vi "Post Test End.vi"(8 "error in (no error)":errorcluster, 9 "Test End Error (no error)":errorcluster, 10 "Test End":enum16{"Normal", "User Abort", "Error"}(ring), 11 "Test":T1) -> (0 "error out":errorcluster)   [LabVIEW 2016, in "Hall Effect Library.lvlib"]
uses:
  Hall Effect Library.lvlib
  Public/Controls/Tests.ctl
  Public/Controls/Message Types.ctl
  Global Variables/Communication.vi
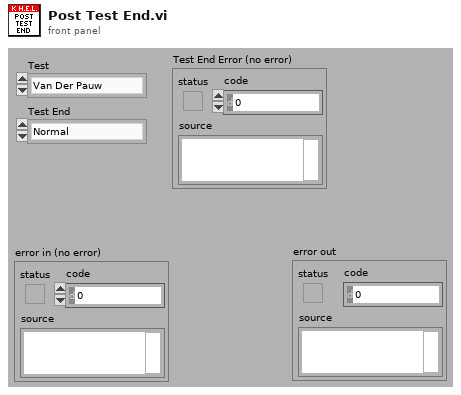
[diagram p1: front panel]
types:
  T1 = typedef "Hall Effect Library.lvlib/Tests.ctl" = enum16{"Van Der Pauw", "Hall Effect", "Bar Sample Resistivity", "Bar Sample Hall ", "6-Contact Sample Resistivity", "6-Contact Sample Hall", "8-Contact Sample Resistivity", "8-Contact Sample Hall", ""}
  T2 = typedef "Hall Effect Library.lvlib/Message Types.ctl" = enum16{"Status", "New Data", "Test End Normal", "Test End User Abort", "Test End Error"}
  T3 = cluster{"Test":T1, "Test End Error (no error)":errorcluster}
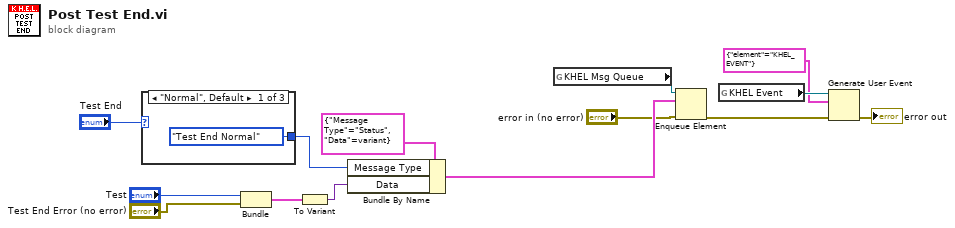
[diagram p0: block diagram]
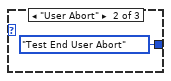
[diagram p2: hidden frame]
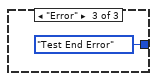
[diagram p3: hidden frame]
diagram:
  n1 = case shown="\"Normal\", Default" "Test End" {
    tunnel: [Message_Types."Test End Normal" ("Message Type") Message_Types."Test End User Abort" ("Message Type") Message_Types."Test End Error" ("Message Type")] -> w12
    frame "Normal", Default {
    }
    frame "User Abort" {
    }
    frame "Error" {
    }
  }
  n2 = Bundle("Test"="Test", "Test End Error (no error)"="Test End Error (no error)") -> (w7:T3)  [unwired: 1 out]
  n3 = To Variant(anything=w7) -> (Variant=w11:variant)
  n4 = Bundle By Name(cluster=cluster{"Message Type":T2, "Data":variant} {"Message Type"=enum."Status", "Data"=variant} ("element"), "Message Type"=w12, "Data"=w11) -> (w10:cluster{"Message Type":T2, "Data":variant})
  n5 = global read "Communication.vi" "KHEL Msg Queue"() -> (w14:refnum<queue>)
  n6 = Enqueue Element(queue=w14, element=w10, error in (no error)="error in (no error)") -> (error out=w3:errorcluster)  [unwired: 3 out]
  n7 = global read "Communication.vi" "KHEL Event"() -> (w2:refnum<user-event>)
  n8 = Generate User Event(user event=w2, event data cluster=cluster{"element":string} {"element"="KHEL_EVENT"}, error in=w3) -> (error out=→"error out":errorcluster)  [unwired: 1 in, 1 out]
